vi "getAdditionalDataFromXML.vi"(8 "error in (no error)":errorcluster, 10 "Xml":refnum<class "xmlNode.lvclass">, 11 "SingleTone in":refnum<class "SingleTone.lvclass">) -> (0 "error out":errorcluster, 2 "Xml out":refnum<class "xmlNode.lvclass">, 3 "SingleTone out":refnum<class "SingleTone.lvclass">)   [LabVIEW 2009, in "Tools.lvlib" / "Scripting.lvlib" / "SingleTone.lvclass"]
uses:
  SingleTone.lvclass
  xmlNode/xmlNode.lvclass
  SingleToneArray/SingleToneArray.lvclass
  SingleTone.lvclass/SingleTone.ctl
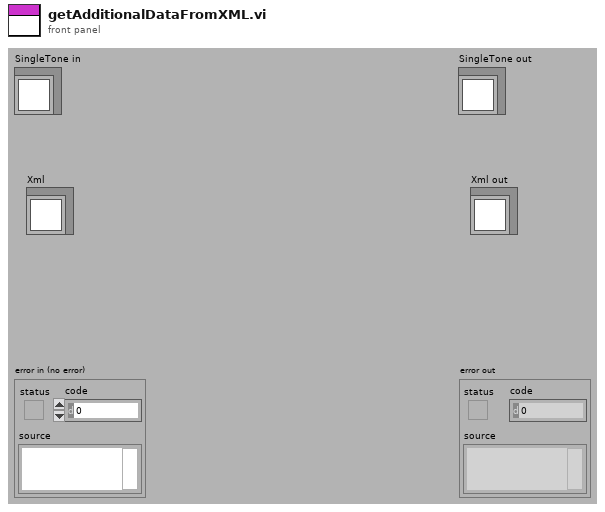
[diagram p1: front panel]
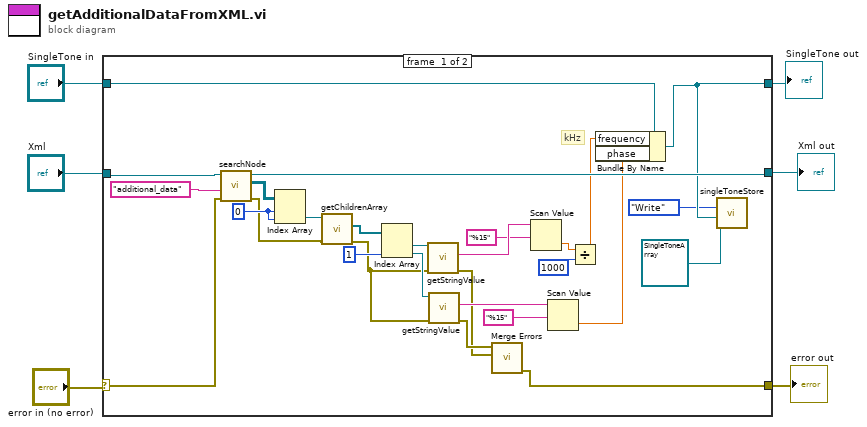
[diagram p0: block diagram]
diagram:
  n1 = case shown="No Error" "error in (no error)" {
    selector: "error in (no error)" -> [w19 w35]
    tunnel: "SingleTone in" -> [w22 w37]
    tunnel: [w9 w37] -> w5
    tunnel: [w28 w36] -> w4
    tunnel: "Xml" -> [w27 w36]
    tunnel: [w10 w35] -> w1
    frame #0 {
      w33 = 0
      # "kHz"
      n2 = call-dynamic "searchNode.vi"("error in (no error)"=w19, "searchElementName"="additional_data", "xmlNode in"=w27) -> ("error out"=w31:errorcluster, "arrayXmlNodes"=w34:refnum<class "xmlNode.lvclass">[][], "xmlNode out"=w28:refnum<class "xmlNode.lvclass">)  [unwired: 6 in]
      n3 = Index Array(array=w34, index (row)=w33, index (col)=w33) -> (element=w32:refnum<class "xmlNode.lvclass">)
      n4 = call-dynamic "getChildrenArray.vi"("error in (no error)"=w31, "xmlNode.lvclass in"=w32) -> ("error out"=w16:errorcluster, "Children"=w30:refnum<class "xmlNode.lvclass">[])  [unwired: 7 in, 1 out]
      n5 = Index Array(array=w30, index #2=1) -> (element #1=w29:refnum<class "xmlNode.lvclass">, element #2=w17:refnum<class "xmlNode.lvclass">)  [unwired: 1 in]
      n6 = call-dynamic "getStringValue.vi"("error in (no error)"=w16, "xmlNode.lvclass in"=w29) -> ("error out"=w11:errorcluster, "stringValue"=w26:string)  [unwired: 7 in, 1 out]
      n7 = call-dynamic "getStringValue.vi"("error in (no error)"=w16, "xmlNode.lvclass in"=w17) -> ("error out"=w12:errorcluster, "stringValue"=w14:string)  [unwired: 7 in, 1 out]
      n8 = call <vilib>:"Merge Errors.vi"("error in 2 (no error)"=w11, "error in 1 (no error)"=w12) -> ("error out"=w10:errorcluster)  [unwired: 5 in]
      n9 = Scan Value(string=w26, format string="%15") -> (value=w24:dbl)  [unwired: 1 in, 1 out]
      n10 = Scan Value(string=w14, format string="%15") -> (value=w13:dbl)  [unwired: 1 in, 1 out]
      n11 = Divide(x=w24, y=1000) -> (x/y=w21:dbl)
      n12 = Bundle By Name(cluster=w22, "frequency"=w21, "phase"=w13) -> (w9:refnum<class "SingleTone.lvclass">)
      n13 = call "singleToneStore.vi"("SingleTone.lvclass"=w9, "action"=enum16{"Write", "Read"}."Write", "SingleToneArray in"=refnum<class "SingleToneArray.lvclass"> refnum) -> ()  [unwired: 5 in, 4 out]
    }
    frame #1 {
    }
  }
  "error out" <- w1
  "SingleTone out" <- w5
  "Xml out" <- w4
